vi "AerotechGUI.vi"() -> ()   [LabVIEW 2009, in "Aerotech.lvlib"]
uses:
  Aerotech.lvlib
  Controls/AerotechTarget.ctl
  Controls/AerotechState.ctl
panel:
  out "State":T1
  out "AEROTECH.TARGET":T2
  in  "Position":dbl
  in  "POSITION Button":bool
  in  "HOME button":bool
  in  "IDLE Button":bool
  in  "TRACK Button":bool
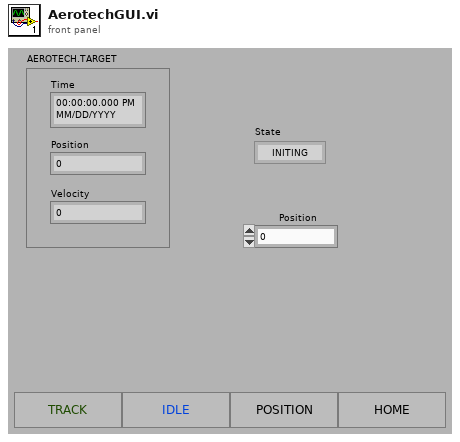
[diagram p1: front panel]
types:
  T1 = typedef "AerotechState.ctl" = enum16{"INITING", "IDLING", "SLEWING", "TRACKING", "MOVING", "HOMING", "STOPPING"}
  T2 = typedef "AerotechTarget.ctl" = cluster{"Time":timestamp, "Position":dbl, "Velocity":dbl}
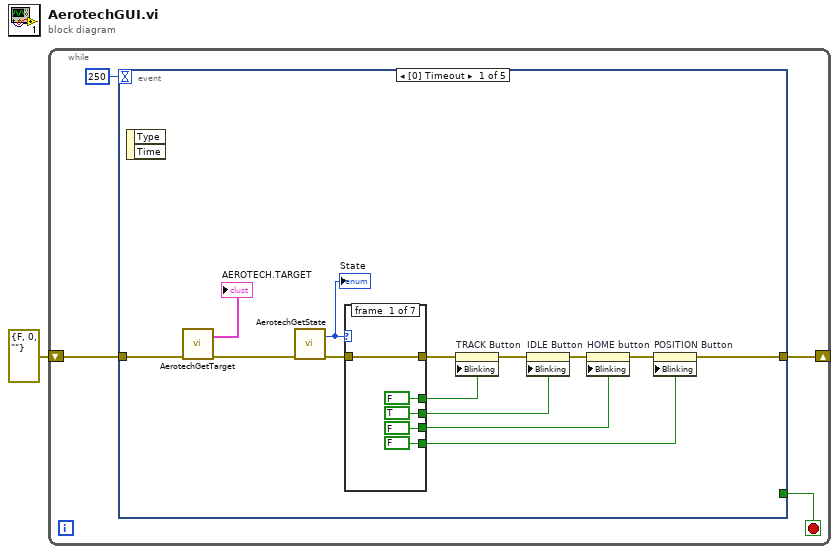
[diagram p0: block diagram]
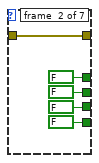
[diagram p2: hidden frame]
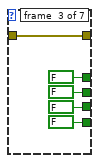
[diagram p3: hidden frame]
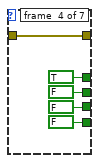
[diagram p4: hidden frame]
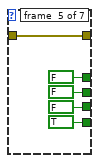
[diagram p5: hidden frame]
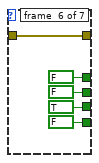
[diagram p6: hidden frame]
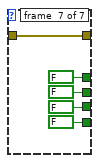
[diagram p7: hidden frame]
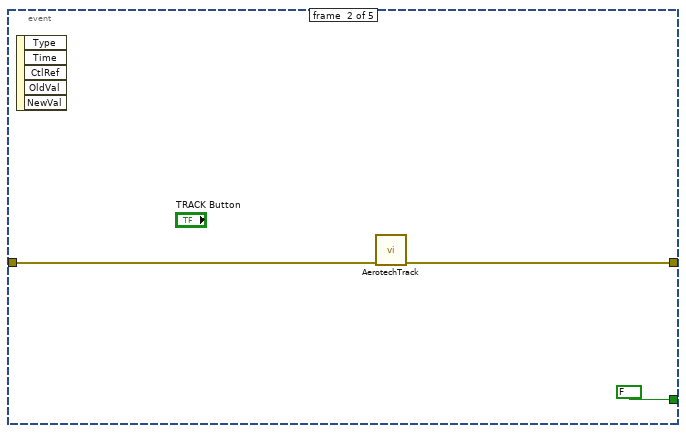
[diagram p8: hidden frame]
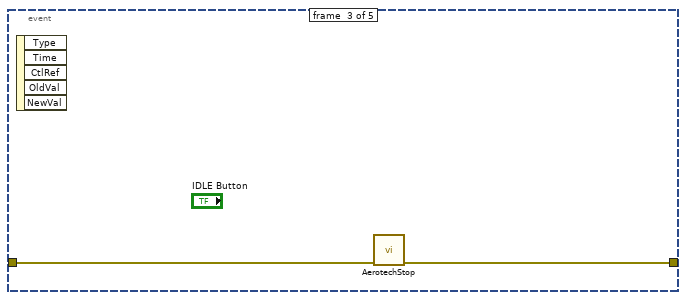
[diagram p9: hidden frame]
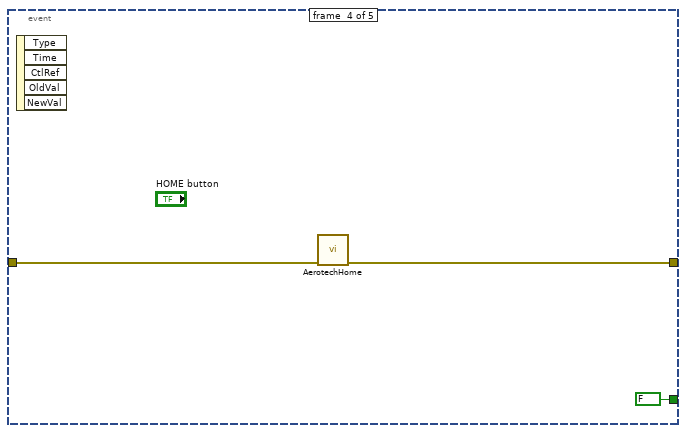
[diagram p10: hidden frame]
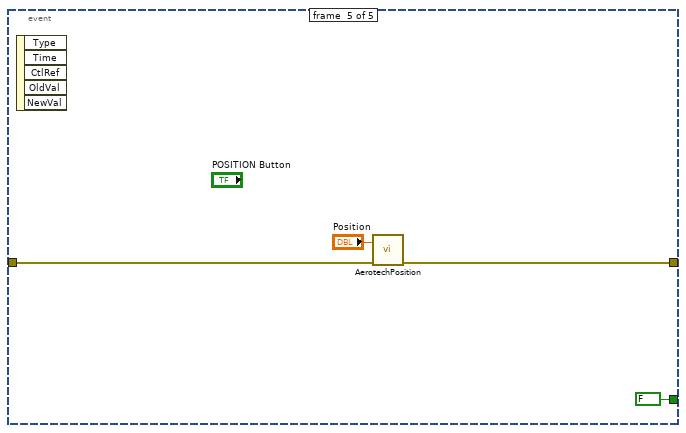
[diagram p11: hidden frame]
diagram:
  n1 = while {
    shift-right: [w4] -> _
    shift-left: errorcluster {"status"=FALSE, "code"=0, "source"=""} ("error out") -> [w5]
    stop <- w2 stop-if-true
    n2 = event shown="[0] Timeout" {
      selector: _ -> [_ _ _ _ _]
      dyn-events: _ -> [_ _ _ _ _]
      timeout: 250 -> [_ _ _ _ _]
      tunnel: w5 -> [w9 w57 w59 w62 w66]
      tunnel: [w16 w56 w58 w61 w65] -> w4
      tunnel: [_ FALSE _ FALSE FALSE] -> w2
      event #0 {
        n3 = event-data() -> ()  [unwired: 1 in, 2 out]
        n4 = call "AerotechGetTarget.vi"("error in (no error)"=w9) -> ("error out"=w8:errorcluster, "AEROTECH.TARGET"=→"AEROTECH.TARGET":T2)  [unwired: 3 in]
        n5 = call "AerotechGetState.vi"("error in (no error)"=w8) -> ("error out"=w15:errorcluster, "State"=w6:T1)  [unwired: 3 in]
        "State" <- w6
        n6 = case shown="\"HOMING\"" w6 {
          tunnel: w15 -> [w24 w29 w34 w39 w44 w49 w54]
          tunnel: [w24 w29 w34 w39 w44 w49 w54] -> w14
          tunnel: [FALSE FALSE FALSE TRUE FALSE FALSE FALSE] -> w13
          tunnel: [TRUE FALSE FALSE FALSE FALSE FALSE FALSE] -> w12
          tunnel: [FALSE FALSE FALSE FALSE FALSE TRUE FALSE] -> w11
          tunnel: [FALSE FALSE FALSE FALSE TRUE FALSE FALSE] -> w10
          frame #0 {
          }
          frame #1 {
          }
          frame #2 {
          }
          frame #3 {
          }
          frame #4 {
          }
          frame #5 {
          }
          frame #6 {
          }
        }
        n7 = property on="TRACK Button" class="Bool"(error in=w14, "Blinking"=w13) -> (error out=w19:errorcluster)  [unwired: 1 in, 1 out]
        n8 = property on="IDLE Button" class="Bool"(error in=w19, "Blinking"=w12) -> (error out=w18:errorcluster)  [unwired: 1 in, 1 out]
        n9 = property on="HOME button" class="Bool"(error in=w18, "Blinking"=w11) -> (error out=w17:errorcluster)  [unwired: 1 in, 1 out]
        n10 = property on="POSITION Button" class="Bool"(error in=w17, "Blinking"=w10) -> (error out=w16:errorcluster)  [unwired: 1 in, 1 out]
      }
      event #1 {
        n11 = event-data() -> ()  [unwired: 1 in, 5 out]
        n12 = call "AerotechTrack.vi"("error in (no error)"=w57) -> ("error out"=w56:errorcluster)  [unwired: 10 in]
      }
      event #2 {
        n13 = event-data() -> ()  [unwired: 1 in, 5 out]
        n14 = call "AerotechStop.vi"("error in (no error)"=w59) -> ("error out"=w58:errorcluster)  [unwired: 10 in]
      }
      event #3 {
        n15 = event-data() -> ()  [unwired: 1 in, 5 out]
        n16 = call "AerotechHome.vi"("error in (no error)"=w62) -> ("error out"=w61:errorcluster)  [unwired: 10 in]
      }
      event #4 {
        n17 = event-data() -> ()  [unwired: 1 in, 5 out]
        n18 = call "AerotechPosition.vi"("error in (no error)"=w66, "Position"="Position") -> ("error out"=w65:errorcluster)  [unwired: 3 in]
      }
    }
  }
